vi "BP Set Properties.vi"(8 "error in":errorcluster, 10 "View Model in":T1, 11 "TDMS in":refnum<class "TDMS.lvclass">) -> (0 "error out":errorcluster, 3 "TDMS out":refnum<class "TDMS.lvclass">)   [LabVIEW 2017, in "Report_lib.lvlib" / "TDMS.lvclass"]
doc: "This SubVI set Gpoups\\Channels properties\nduring creation of TDMS file"
uses:
  TDMS.lvclass
  View Model/Controls/View Model.ctl
  View Model/Controls/Shared Model.ctl
  Error Handler/Controls/Error Model.ctl
  Error Handler/Controls/Error Event.ctl
  Error Handler/Controls/Error Type.ctl
  Controller/Controls/Controller Model.ctl
  Controller/Controls/Controller Event.ctl
  Controller/Controls/Controller Command.ctl
  Controller/Controls/Controller Overhead.ctl
  Real-Time/RT Status.ctl
  Real-Time/RT Loop Status.ctl
  Controller/Controls/Controller NStream.ctl
  Controller/Controls/Controller DAQ Data.ctl
  TDMS Logger/Controls/TDMS Model.ctl
  TDMS Logger/Controls/TDMS Event.ctl
  TDMS Logger/Controls/TDMS Command.ctl
  TDMS Logger/Controls/TDMS Overhead.ctl
  TDMS Logger/Controls/TDMS ChanProperties.ctl
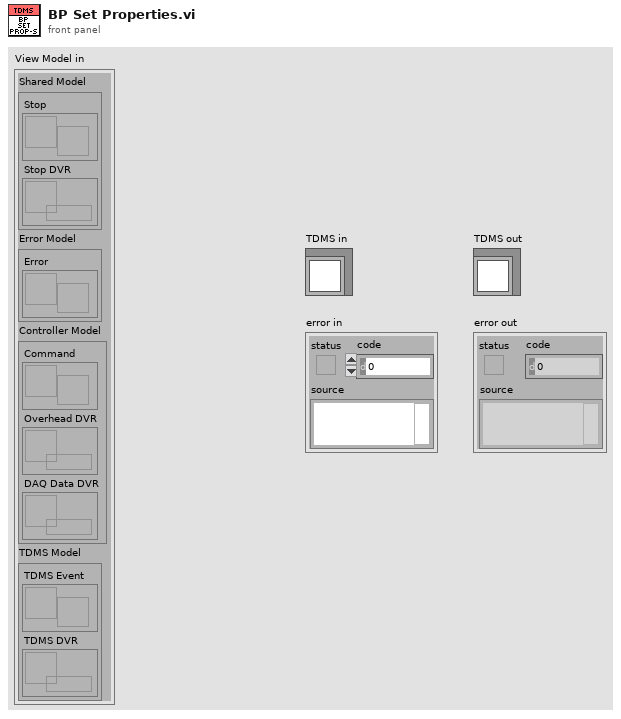
[diagram p1: front panel]
types:
  T1 = typedef "View Model.ctl" = cluster{"Shared Model":T2, "Error Model":T3, "Controller Model":T4, "TDMS Model":T5}
  T2 = typedef "Shared Model.ctl" = cluster{"Stop":refnum<user-event>, "Stop DVR":refnum<data-value>}
  T3 = typedef "Error Model.ctl" = cluster{"Error":refnum<user-event>}
  T4 = typedef "Controller Model.ctl" = cluster{"Command":refnum<user-event>, "Overhead DVR":refnum<data-value>, "DAQ Data DVR":refnum<data-value>}
  T5 = typedef "TDMS Model.ctl" = cluster{"TDMS Event":refnum<user-event>, "TDMS DVR":refnum<data-value>}
  T6 = typedef "TDMS ChanProperties.ctl" = cluster{"AOM9":string[][], "AIM2":string[][], "DIM3":string[][], "DIM4":string[][], "DOM6":string[][], "DOM7":string[][]}
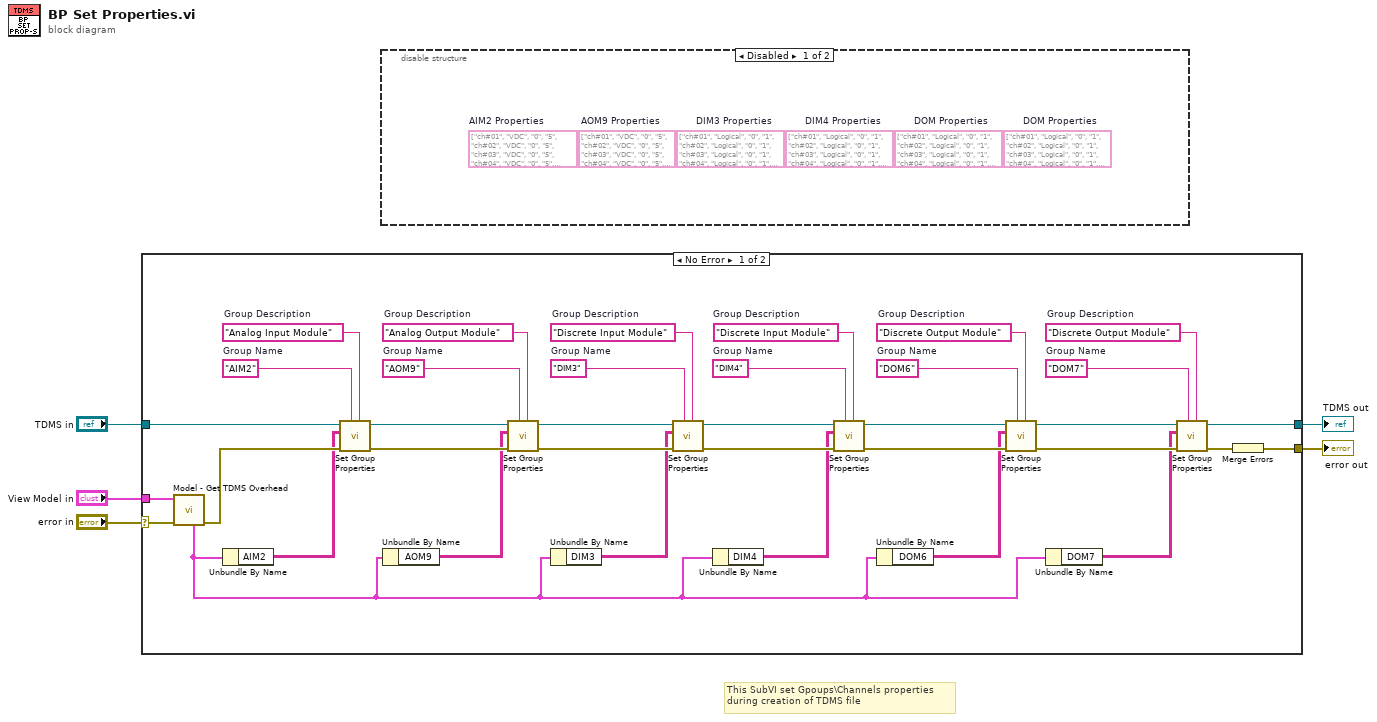
[diagram p0: block diagram]
diagram:
  # "This SubVI set Gpoups\\Channels properties\nduring creation of TDMS file"
  n1 = case shown="No Error" "error in" {
    selector: "error in" -> [w40 w43]
    tunnel: [w12 w43] -> w4
    tunnel: [w14 w42] -> w2
    tunnel: "TDMS in" -> [w36 w42]
    tunnel: "View Model in" -> [w41 _]
    frame No Error {
      w37 = "Analog Output Module"  # Group Description
      w38 = "AOM9"  # Group Name
      w16 = "Discrete Output Module"  # Group Description
      w15 = "DOM7"  # Group Name
      w20 = "Discrete Output Module"  # Group Description
      w19 = "DOM6"  # Group Name
      w23 = "Discrete Input Module"  # Group Description
      w24 = "DIM4"  # Group Name
      w28 = "Discrete Input Module"  # Group Description
      w27 = "DIM3"  # Group Name
      w31 = "Analog Input Module"  # Group Description
      w32 = "AIM2"  # Group Name
      n2 = call "Model - Get TDMS Overhead.vi"("error in (no error)"=w40, "View Model"=w41) -> ("error out"=w35:errorcluster, "ChProps"=w39:T6)  [unwired: 4 in, 4 out]
      n3 = Unbundle By Name(w39) -> ("AIM2"=w11:string[][])
      n4 = call "Set Group Properties.vi"("Group Description"=w31, "Group Name"=w32, "error in (no error)"=w35, "Channel Names + Properties"=w11, "TDMS in"=w36) -> ("error out"=w34:errorcluster, "TDMS out"=w33:refnum<class "TDMS.lvclass">)  [unwired: 5 in]
      n5 = Unbundle By Name(w39) -> ("AOM9"=w10:string[][])
      n6 = call "Set Group Properties.vi"("Group Description"=w37, "Group Name"=w38, "error in (no error)"=w34, "Channel Names + Properties"=w10, "TDMS in"=w33) -> ("error out"=w30:errorcluster, "TDMS out"=w29:refnum<class "TDMS.lvclass">)  [unwired: 5 in]
      n7 = Unbundle By Name(w39) -> ("DIM3"=w9:string[][])
      n8 = call "Set Group Properties.vi"("Group Description"=w28, "Group Name"=w27, "error in (no error)"=w30, "Channel Names + Properties"=w9, "TDMS in"=w29) -> ("error out"=w26:errorcluster, "TDMS out"=w25:refnum<class "TDMS.lvclass">)  [unwired: 5 in]
      n9 = Unbundle By Name(w39) -> ("DIM4"=w8:string[][])
      n10 = call "Set Group Properties.vi"("Group Description"=w23, "Group Name"=w24, "error in (no error)"=w26, "Channel Names + Properties"=w8, "TDMS in"=w25) -> ("error out"=w22:errorcluster, "TDMS out"=w21:refnum<class "TDMS.lvclass">)  [unwired: 5 in]
      n11 = Unbundle By Name(w39) -> ("DOM6"=w7:string[][])
      n12 = call "Set Group Properties.vi"("Group Description"=w20, "Group Name"=w19, "error in (no error)"=w22, "Channel Names + Properties"=w7, "TDMS in"=w21) -> ("error out"=w18:errorcluster, "TDMS out"=w17:refnum<class "TDMS.lvclass">)  [unwired: 5 in]
      n13 = Unbundle By Name(w39) -> ("DOM7"=w6:string[][])
      n14 = call "Set Group Properties.vi"("Group Description"=w16, "Group Name"=w15, "error in (no error)"=w18, "Channel Names + Properties"=w6, "TDMS in"=w17) -> ("error out"=w13:errorcluster, "TDMS out"=w14:refnum<class "TDMS.lvclass">)  [unwired: 5 in]
      n15 = Merge Errors(w13) -> (w12:errorcluster)
    }
    frame Error {
    }
  }
  "error out" <- w4
  "TDMS out" <- w2
  n16 = disable-structure shown="Disabled" {
    frame Disabled {
      (unwired) string[][] [["ch#01", "VDC", "0", "5"], ["ch#02", "VDC", "0", "5"], ["ch#03", "VDC", "0", "5"], ["ch#04", "VDC", "0", "5"], ["ch#05", "VDC", "0", "5"], ["ch#06", "VDC", "0", "5"], ["ch#07", "VDC", "0", "5"], ["ch#08", "VDC", "0", "5"], ["ch#09", "VDC", "-", "-"], ["ch#10", "VDC", "-", "-"], ["ch#11", "VDC", "-", "-"], ["ch#12", "VDC", "-", "-"], ["ch#13", "VDC", "-", "-"], ["ch#14", "VDC", "-", "-"], ["ch#15", "VDC", "-", "-"], ["ch#16", "VDC", "-", "-"], ["ch#17", "VDC", "0", "5"], ["ch#18", "VDC", "0", "5"], ["ch#19", "VDC", "0", "5"], ["ch#20", "VDC", "0", "5"], ["ch#21", "VDC", "-", "-"], ["ch#22", "VDC", "-", "-"], ["TimeStamp", "seconds", "", ""]]  # AIM2 Properties
      (unwired) string[][] [["ch#01", "VDC", "0", "5"], ["ch#02", "VDC", "0", "5"], ["ch#03", "VDC", "0", "5"], ["ch#04", "VDC", "0", "5"], ["ch#05", "VDC", "0", "5"], ["ch#06", "VDC", "0", "5"], ["TimeStamp", "seconds", "", ""]]  # AOM9 Properties
      (unwired) string[][] [["ch#01", "Logical", "0", "1"], ["ch#02", "Logical", "0", "1"], ["ch#03", "Logical", "0", "1"], ["ch#04", "Logical", "0", "1"], ["ch#05", "Logical", "0", "1"], ["ch#06", "Logical", "0", "1"], ["ch#07", "Logical", "0", "1"], ["ch#08", "Logical", "0", "1"], ["ch#09", "Logical", "0", "1"], ["ch#10", "Logical", "0", "1"], ["ch#11", "Logical", "0", "1"], ["ch#12", "Logical", "0", "1"], ["ch#13", "Logical", "0", "1"], ["ch#14", "Logical", "0", "1"], ["ch#15", "Logical", "0", "1"], ["ch#16", "Logical", "0", "1"], ["TimeStamp", "seconds", "", ""]]  # DOM Properties
      (unwired) string[][] [["ch#01", "Logical", "0", "1"], ["ch#02", "Logical", "0", "1"], ["ch#03", "Logical", "0", "1"], ["ch#04", "Logical", "0", "1"], ["ch#05", "Logical", "0", "1"], ["ch#06", "Logical", "0", "1"], ["ch#07", "Logical", "0", "1"], ["ch#08", "Logical", "0", "1"], ["ch#09", "Logical", "0", "1"], ["ch#10", "Logical", "0", "1"], ["ch#11", "Logical", "0", "1"], ["ch#12", "Logical", "0", "1"], ["ch#13", "Logical", "0", "1"], ["ch#14", "Logical", "0", "1"], ["ch#15", "Logical", "0", "1"], ["ch#16", "Logical", "0", "1"], ["TimeStamp", "seconds", "", ""]]  # DOM Properties
      (unwired) string[][] [["ch#01", "Logical", "0", "1"], ["ch#02", "Logical", "0", "1"], ["ch#03", "Logical", "0", "1"], ["ch#04", "Logical", "0", "1"], ["ch#05", "Logical", "0", "1"], ["ch#06", "Logical", "0", "1"], ["ch#07", "Logical", "0", "1"], ["ch#08", "Logical", "0", "1"], ["ch#09", "Logical", "0", "1"], ["ch#10", "Logical", "0", "1"], ["ch#11", "Logical", "0", "1"], ["ch#12", "Logical", "0", "1"], ["ch#13", "Logical", "0", "1"], ["ch#14", "Logical", "0", "1"], ["ch#15", "Logical", "0", "1"], ["ch#16", "Logical", "0", "1"], ["ch#17", "Logical", "0", "1"], ["ch#18", "Logical", "0", "1"], ["ch#19", "Logical", "0", "1"], ["ch#20", "Logical", "0", "1"], ["ch#21", "Logical", "0", "1"], ["ch#22", "Logical", "0", "1"], ["ch#23", "Logical", "0", "1"], ["ch#24", "Logical", "0", "1"], ["ch#25", "Logical", "0", "1"], ["ch#26", "Logical", "0", "1"], ["ch#27", "Logical", "0", "1"], ["ch#28", "Logical", "0", "1"], ["ch#29", "Logical", "0", "1"], ["ch#30", "Logical", "0", "1"], ["ch#31", "Logical", "0", "1"], ["ch#32", "Logical", "0", "1"], ["TimeStamp", "seconds", "", ""]]  # DIM4 Properties
      (unwired) string[][] [["ch#01", "Logical", "0", "1"], ["ch#02", "Logical", "0", "1"], ["ch#03", "Logical", "0", "1"], ["ch#04", "Logical", "0", "1"], ["ch#05", "Logical", "0", "1"], ["ch#06", "Logical", "0", "1"], ["ch#07", "Logical", "0", "1"], ["ch#08", "Logical", "0", "1"], ["ch#09", "Logical", "0", "1"], ["ch#10", "Logical", "0", "1"], ["ch#11", "Logical", "0", "1"], ["ch#12", "Logical", "0", "1"], ["ch#13", "Logical", "0", "1"], ["ch#14", "Logical", "0", "1"], ["ch#15", "Logical", "0", "1"], ["ch#16", "Logical", "0", "1"], ["ch#17", "Logical", "0", "1"], ["ch#18", "Logical", "0", "1"], ["ch#19", "Logical", "0", "1"], ["ch#20", "Logical", "0", "1"], ["ch#21", "Logical", "0", "1"], ["ch#22", "Logical", "0", "1"], ["ch#23", "Logical", "0", "1"], ["ch#24", "Logical", "0", "1"], ["ch#25", "Logical", "0", "1"], ["ch#26", "Logical", "0", "1"], ["TimeStamp", "seconds", "", ""]]  # DIM3 Properties
    }
    frame Enabled {
    }
  }
